vi "Create Hyperlink Folders.vi"(0 "Work Sheet":refnum<k7>, 5 "error in":errorcluster) -> (19 "error out":errorcluster)   [LabVIEW 2017]
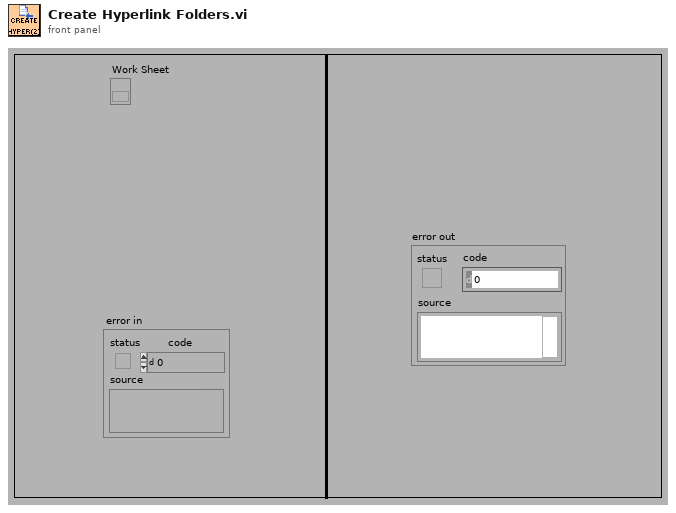
[diagram p1: front panel]
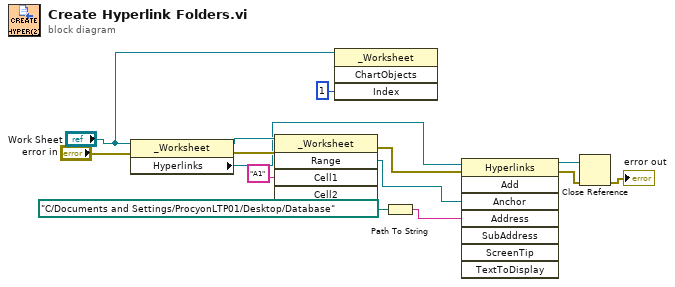
[diagram p0: block diagram]
diagram:
  n1 = property class="_Worksheet"(reference="Work Sheet", error in="error in") -> (reference out=w14:refnum<k7>, error out=w13:errorcluster, "Hyperlinks"=w12:refnum<k7>)
  n2 = invoke class="_Worksheet" method="Range"(reference=w14, error in=w13, "Cell1"="A1" ("Link Cell 1")) -> (error out=w3:errorcluster, "Range"=w11:refnum<k7>)  [unwired: 2 in, 3 out]
  n3 = invoke class="_Worksheet" method="ChartObjects"(reference="Work Sheet", "Index"=1) -> ()  [unwired: 2 in, 4 out]
  n4 = Path To String(path=path "C:/Documents and Settings/ProcyonLTP01/Desktop/Database" ("File Path")) -> (string=w4:string)
  n5 = invoke class="Hyperlinks" method="Add"(reference=w12, error in=w3, "Anchor"=w11, "Address"=w4) -> (reference out=w7:refnum<k7>, error out=w6:errorcluster)  [unwired: 4 in, 6 out]
  n6 = Close Reference(reference=w7, error in (no error)=w6) -> (error out=→"error out":errorcluster)
